vi "Init.vi"(0 "VisaCluster":T1, 11 "error in (no error)":errorcluster) -> (4 "VisaCluster":T1, 8 "Answer":string, 15 "error out":errorcluster)   [LabVIEW 2014, in "FH 55.lvlib"]
doc: "Durch das VI init wird das Gerät neu initalisiert\n\nThe VI initializes the device"
uses:
  FH 55.lvlib
  TypeDef/VisaCluster.ctl
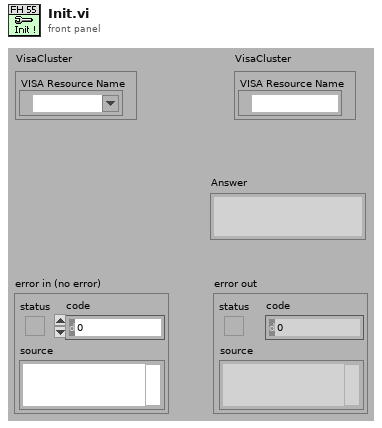
[diagram p1: front panel]
types:
  T1 = typedef "FH 55.lvlib/VisaCluster.ctl" = cluster{"VISA Resource Name":refnum<visa-resource-name>}
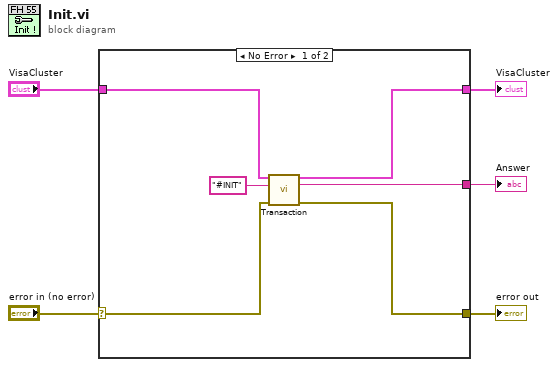
[diagram p0: block diagram]
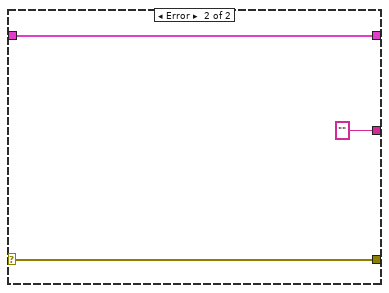
[diagram p2: hidden frame]
diagram:
  n1 = case shown="No Error" "error in (no error)" {
    selector: "error in (no error)" -> [w10 w13]
    tunnel: "VisaCluster" -> [w11 w14]
    tunnel: [w7 w14] -> w1
    tunnel: [w6 w13] -> w3
    tunnel: [w8 ""] -> w2
    frame No Error {
      n2 = call "Transaction.vi"("VisaCluster"=w11, "Command"="#INIT", "error in (no error)"=w10) -> ("VisaCluster"=w7:T1, "Answer"=w8:string, "error out"=w6:errorcluster)  [unwired: 9 in, 1 out]
    }
    frame Error {
    }
  }
  "error out" <- w3
  "Answer" <- w2
  "VisaCluster" <- w1
